vi "Poly_ForStart.vi"   [LabVIEW 2012]
doc: "Begins the execution of a for loop. The loop will execute the specified number of \"iterations\".\nNote: requires Loop end VI."
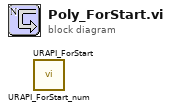
[diagram p0: block diagram]
diagram:
  n1 = call <userlib>:"URAPI_ForStart_num.vi"() -> ()  [unwired: 4 in, 2 out]
  n2 = call <userlib>:"URAPI_ForStart.vi"() -> ()  [unwired: 4 in, 2 out]
